vi "Remove Zero Coefficients.vi"   [LabVIEW 2020, in "NI_AALPro.lvlib"]
doc: "Removes from <B>P(x) In</B> the trailing coefficients near zero whose absolute values are less than <B>threshold</B>. Wire data to the <B>P(x) In</B> input to determine the polymorphic instance to use or manually select the instance."
uses:
  NI_AALPro.lvlib
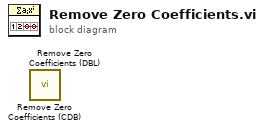
[diagram p0: block diagram]
diagram:
  n1 = call "Remove Zero Coefficients (CDB).vi"() -> ()  [unwired: 9 in, 3 out]
  n2 = call "Remove Zero Coefficients (DBL).vi"() -> ()  [unwired: 9 in, 3 out]
